vi "read AI 1D.vi"(8 "error in (no error)":errorcluster, 9 "timeout (s)":dbl=10.0 format="%0.2f", 10 "number of samples per channel":i32=-1, 11 "Refnum in":refnum<k21>) -> (0 "error out":errorcluster, 2 "data":waveform(dbl)[](array[waveform]), 3 "Refnum out":refnum<k21>)   [LabVIEW 2018]
uses:
  <vilib>/DAQmx/read.llb/DAQmx Read.vi
  <vilib>/DAQmx/read.llb/DAQmx Read (Analog 1D Wfm NChan NSamp).vi
  <vilib>/DAQmx/miscellaneous.llb/DAQmx Fill In Error Info.vi
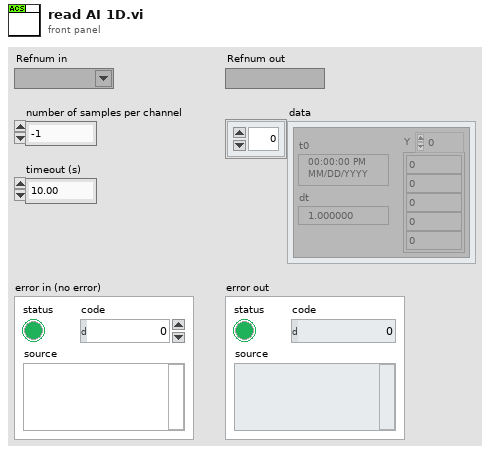
[diagram p1: front panel]
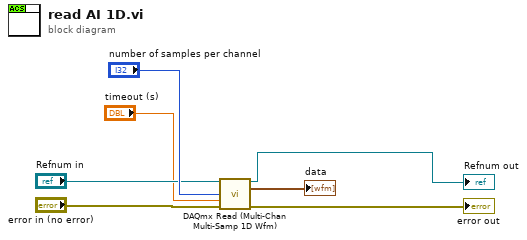
[diagram p0: block diagram]
diagram:
  n1 = call-poly "DAQmx Read (Multi-Chan Multi-Samp 1D Wfm).vi"("task/channels in"="Refnum in", "number of samples per channel"="number of samples per channel", "timeout"="timeout (s)", "error in"="error in (no error)") -> ("task out"=→"Refnum out":refnum<k21>, "data"=→"data":waveform(dbl)[], "error out"=→"error out":errorcluster)  [unwired: 9 in]
